vi "Read Server Internal UEs.vi"(8 "error in (no error)":errorcluster, 11 "gRPC service in":refnum<class "PluginLoader.lvclass">) -> (0 "error out":errorcluster, 2 "Server Internal UEs":T1, 3 "gRPC service out":refnum<class "PluginLoader.lvclass">)   [LabVIEW 2021, in "CIF_PluginLoader_server.lvlib" / "PluginLoader.lvclass"]
uses:
  PluginLoader.lvclass
  typeDefs/Server Internal UEs.ctl
  typeDefs/Server Internal Message.ctl
  PluginLoader.lvclass/PluginLoader.ctl
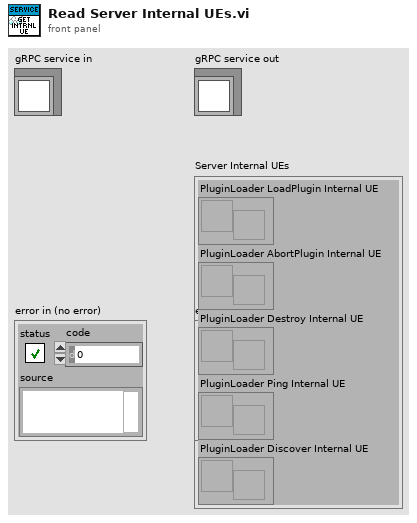
[diagram p1: front panel]
types:
  T1 = typedef "CIF_PluginLoader_server.lvlib/PluginLoader.lvclass/Server Internal UEs.ctl" = cluster{"PluginLoader LoadPlugin Internal UE":refnum<user-event>, "PluginLoader AbortPlugin Internal UE":refnum<user-event>, "PluginLoader Destroy Internal UE":refnum<user-event>, "PluginLoader Ping Internal UE":refnum<user-event>, "PluginLoader Discover Internal UE":refnum<user-event>}
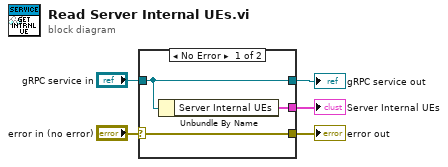
[diagram p0: block diagram]
diagram:
  n1 = case shown="No Error" "error in (no error)" {
    selector: "error in (no error)" -> [w8 w9]
    tunnel: [w8 w9] -> w4
    tunnel: [w7 w10] -> w2
    tunnel: "gRPC service in" -> [w7 w10]
    tunnel: [w6 _] -> w1
    frame No Error {
      n2 = Unbundle By Name(w7) -> ("Server Internal UEs"=w6:T1)
    }
    frame Error {
    }
  }
  "error out" <- w4
  "gRPC service out" <- w2
  "Server Internal UEs" <- w1
